vi "Continuous Serial Read 05.vi"() -> ()   [LabVIEW 2018]
doc: "This example performs writes and reads on a serial port, as directed by the user. You can press the Write and Read buttons, and change the Read Count, while the example is running.\n\nThe parameters set for the serial port must match the parameters of the connected instrument or device. In this example, the Read Count parameter specifies the number of bytes that the serial port reads. If there were more bytes at the port than the specified number, those bytes would not be read. If there were less bytes at the port than the specified number, you would receive a timeout error.\n\nThis example expands upon the flow control options for XON and XOFF, allowing the user to choose those control characters. Also, the user can enable or disable a termination character. Some devices require a termination character in order to identify the end of command strings. Some devices send a termination character to signify the end of data to be read. This example shows how you can end the Read operation once a termination character is detected in the buffer and/or append a termination character at the end of the Write data."
uses:
  <vilib>/Instr/_visa.llb/VISA Configure Serial Port (Instr).vi
panel:
  out "Waveform Chart":dbl(graph)
  out "Sensor Data":dbl
  out "Time (s)":dbl
  in  "file path (use dialog)":path=path "F:/Kerjaan Kantor/Programming/LabVIEW Serial Arduino/1 Ch Sensor/logdata/logsavedata12.txt"
  in  "Baud Rate":u32(ring)=115200 items=["75"=75, "110"=110, "134"=134, "150"=150, "300"=300, "600"=600, "1200"=1200, "1800"=1800, "2400"=2400, "4800"=4800, "7200"=7200, "9600"=9600, "14400"=14400, "19200"=19200, "28800"=28800, "38400"=38400, "56000"=56000, "57600"=57600, "115200"=115200, "128000"=128000, "230400"=230400]
  in  "Stop":bool
  out "Serial Monitor":string
  in  "Serial Port":refnum<visa-resource-name>="COM1"
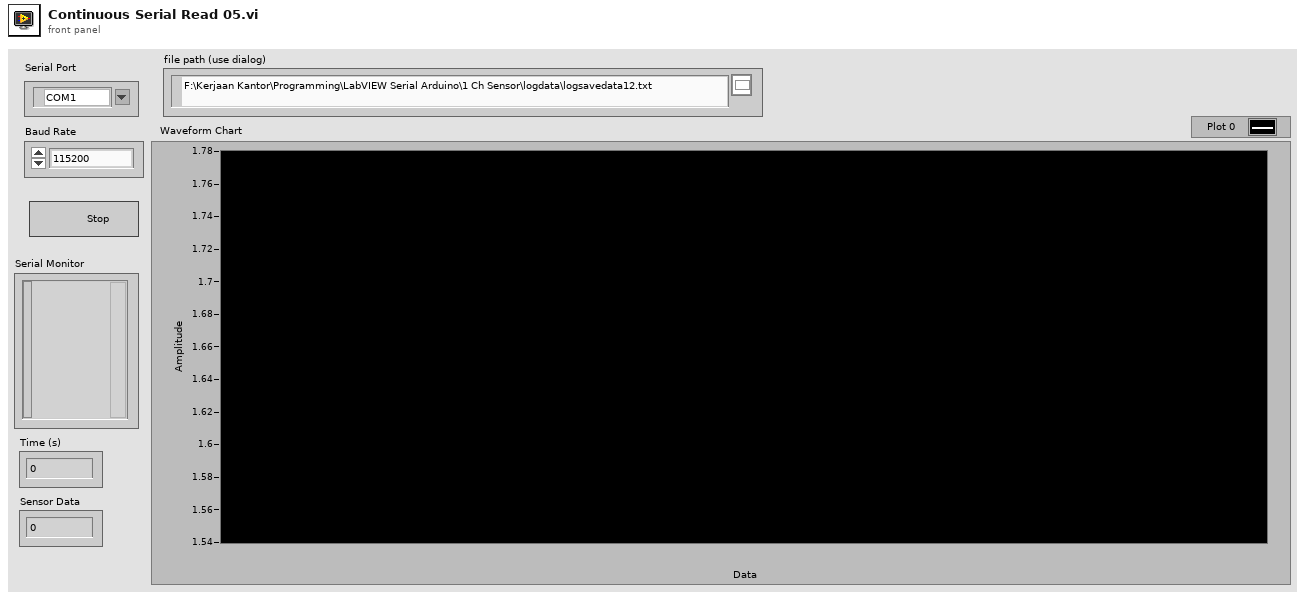
[diagram p1: front panel]
types:
  T1 = enum16{"open", "replace", "create", "open or create", "replace or create", "replace or create with confirmation"}
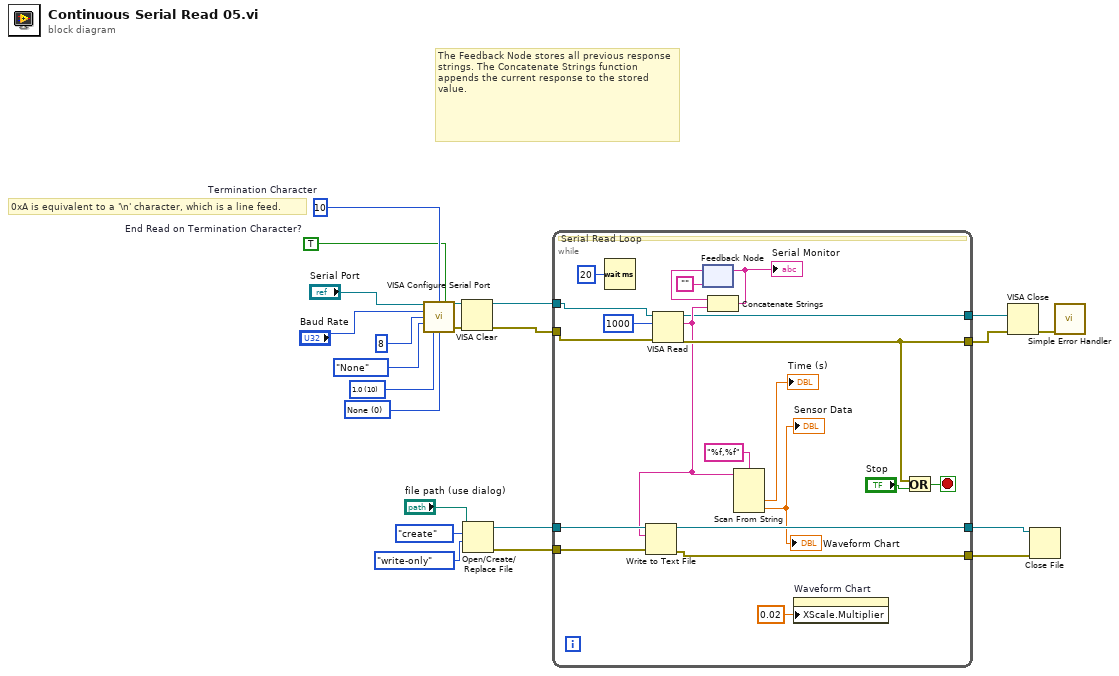
[diagram p0: block diagram]
diagram:
  w14 = TRUE  # End Read on Termination Character?
  w15 = u8 10  # Termination Character
  w17 = u16 0 items=["None", "XON/XOFF", "RTS/CTS", "XON/XOFF & RTS/CTS", "DTR/DSR", "XON/XOFF & DTR/DSR"] ("flow control (0:none)")
  w18 = u16 10 items=["1.0"=10, "1.5"=15, "2.0"=20] ("stop bits (10: 1 bit)")
  # "The Feedback Node stores all previous response strings. The Concatenate Strings function appends the current response to the stored value."
  # "0xA is equivalent to a '\\n' character, which is a line feed."
  n1 = call-poly "VISA Configure Serial Port"("VISA resource name"="Serial Port", "termination char\n(0xA = '\\n' = LF)"=w15, "Enable Termination\nChar (T)"=w14, "baud rate (9600)"="Baud Rate", "data bits (8)"=u16 8, "parity (0:none)"=enum16{"None", "Odd", "Even", "Mark", "Space"}."None", "stop bits (10: 1 bit)"=w18, "flow control (0:none)"=w17) -> ("VISA resource name out"=w13:refnum<visa-resource-name>, "error out"=w12:errorcluster)  [unwired: 2 in, 4 out]
  n2 = VISA Clear(VISA resource name=w13, error in (no error)=w12) -> (VISA resource name out=w2:refnum<visa-resource-name>, error out=w11:errorcluster)
  n3 = Open/Create/Replace File(file path (use dialog)="file path (use dialog)", operation (0:open)=T1."create", access (0:read/write)=enum16{"read/write", "read-only", "write-only"}."write-only") -> (refnum out=w10:refnum<file>, error out=w9:errorcluster)  [unwired: 3 in, 1 out]
  n4 = while {
    tunnel: w11 -> [w36]
    tunnel: [w35] -> w3
    tunnel: w10 -> [w34]
    tunnel: w9 -> [w33]
    tunnel: [w32] -> w8
    tunnel: [w31] -> w7
    tunnel: w2 -> [w25]
    tunnel: [w24] -> w1
    stop <- w41 stop-if-true
    # "Serial Read Loop"
    n5 = Wait (ms)(milliseconds to wait=u32 20) -> ()  [unwired: 1 out]
    n6 = VISA Read(VISA resource name=w25, byte count=u32 1000 ("Read Count"), error in (no error)=w36) -> (VISA resource name out=w24:refnum<visa-resource-name>, read buffer=w30:string, error out=w35:errorcluster)  [unwired: 1 out]
    n7 = Write to Text File(file (use dialog)=w34, text=w30, error in=w33) -> (refnum out=w32:refnum<file>, error out=w31:errorcluster)  [unwired: 1 in, 1 out]
    n8 = feedback #1("") -> (w39:string)
    n9 = Concatenate Strings(w39, w30) -> (w38:string)
    "Serial Monitor" <- w38
    n10 = feedback-in #1(w38) -> ()
    n11 = Scan From String(format string="%f,%f", input string=w30) -> (output 1=→"Time (s)":dbl, output 2=→"Sensor Data" →"Waveform Chart":dbl)  [unwired: 4 in, 3 out]
    n12 = property on="Waveform Chart" class="WFChart (strict)"("XScale.Multiplier"=0.02 ("X Scale.Offset and Multiplier:Multiplier")) -> ()  [unwired: 2 in, 2 out]
    n13 = Or(x=w35, y="Stop") -> (x .or. y?=w41:bool)
  }
  n14 = VISA Close(VISA resource name=w1, error in (no error)=w3) -> (error out=w21:errorcluster)
  n15 = Close File(refnum=w8, error in=w7) -> ()  [unwired: 2 out]
  n16 = call <vilib>:"Simple Error Handler.vi"("error in (no error)"=w21) -> ()  [unwired: 1 in, 8 out]
